vi "Aeroflex ATT Initialize.vi"(8 "error in (no error)":errorcluster, 11 "Configuration":T2={"BusType"=enum."USB", "Card"=0, "USB"="", "IP"=0, "COM"=1, "Baud Rate"=enum."9600"}) -> (0 "error out":errorcluster {"code" format="%.0x"}, 3 "DAQmx Dev Name (PAModule)":string, 5 "Aeroflex ATT":T1)   [LabVIEW 2011]
uses:
  TypeDefs/Aeroflex ATT Configuration.ctl
  TypeDefs/Aeroflex ATT Instrument Info.ctl
  BPIMCore EXT/WebEngine/LIB/MODULES/PA Module/PA Module Tasks.ctl
  <vilib>/DAQmx/create/channels.llb/DAQmx Create Channel (DO-Digital Output).vi
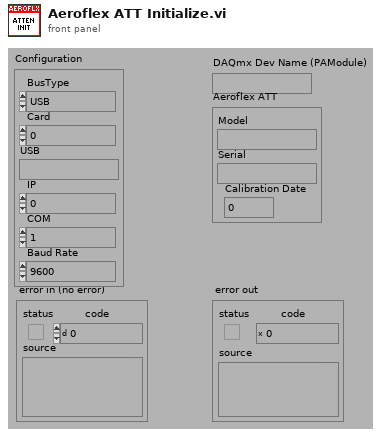
[diagram p1: front panel]
types:
  T1 = typedef "Aeroflex ATT Instrument Info.ctl" = cluster{"Model":string, "Serial":string, "Calibration Date":dbl}
  T2 = typedef "Aeroflex ATT Configuration.ctl" = cluster{"BusType":enum32{"PCI/ISA/PCMCIA", "USB", "Ethernet", "Serial"}, "Card":i32, "USB":string, "IP":u32, "COM":i32, "Baud Rate":enum16{"300", "600", "1200", "2400", "4800", "9600"}}
  T3 = typedef "PA Module Tasks.ctl" = enum16{"PAModule_ID", "PAModule_Alarm", "PAModule_VA1", "PAModule_VA2", "PAModule_SW"}
  T4 = enum32{"PCI/ISA/PCMCIA", "USB", "Ethernet", "Serial"}
  T5 = enum16{"300", "600", "1200", "2400", "4800", "9600"}
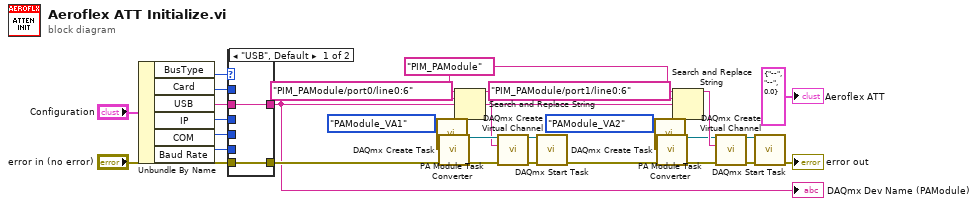
[diagram p0: block diagram]
diagram:
  w1 = "PIM_PAModule" ("DAQmx Dev Name (PIM_PAModule)")
  n1 = Unbundle By Name("Configuration") -> ("BusType"=w29:T4, "Card"=w28:i32, "USB"=w27:string, "IP"=w26:u32, "COM"=w25:i32, "Baud Rate"=w23:T5)
  n2 = case shown="\"USB\", Default" w29 {
    tunnel: "error in (no error)" -> [w32 w33]
    tunnel: w28 -> [_ _]
    tunnel: w27 -> [w31 _]
    tunnel: w26 -> [_ _]
    tunnel: w25 -> [_ _]
    tunnel: [w32 w33] -> w14
    tunnel: [w31 _] -> w4
    tunnel: w23 -> [_ _]
    frame "USB", Default {
    }
    frame "PCI/ISA/PCMCIA", "Ethernet", "Serial" {
    }
  }
  "DAQmx Dev Name (PAModule)" <- w4
  n3 = call "PA Module Task Converter.vi"("PA Module Task"=PA_Module_Tasks."PAModule_VA1" ("RFModule Tasks and Channels")) -> ("Task/Channel Name"=w17:refnum<k21>)  [unwired: 7 out]
  n4 = call <vilib>:"DAQmx Create Task.vi"("new task name"=w17, "error in"=w14) -> ("task out"=w21:refnum<k21>, "error out"=w22:errorcluster)  [unwired: 3 in, 9 out]
  n5 = Search and Replace String(input string=tag "PIM_PAModule/port0/line0:6" ("lines"), search string=w1, replace string=w4) -> (result string=w16:string)  [unwired: 2 in, 6 out]
  n6 = call-poly <vilib>:"DAQmx Create Virtual Channel.vi"("task in"=w21, "lines"=w16, "error in"=w22) -> ("task out"=w19:refnum<k21>, "error out"=w20:errorcluster)  [unwired: 2 in, 9 out]
  n7 = call <vilib>:"DAQmx Start Task.vi"("task/channels in"=w19, "error in"=w20) -> ("error out"=w3:errorcluster)  [unwired: 13 out]
  n8 = call "PA Module Task Converter.vi"("PA Module Task"=PA_Module_Tasks."PAModule_VA2" ("RFModule Tasks and Channels")) -> ("Task/Channel Name"=w10:refnum<k21>)  [unwired: 7 out]
  n9 = call <vilib>:"DAQmx Create Task.vi"("new task name"=w10, "error in"=w3) -> ("task out"=w6:refnum<k21>, "error out"=w5:errorcluster)  [unwired: 3 in, 9 out]
  n10 = Search and Replace String(input string=tag "PIM_PAModule/port1/line0:6" ("lines"), search string=w1, replace string=w4) -> (result string=w11:string)  [unwired: 2 in, 6 out]
  n11 = call-poly <vilib>:"DAQmx Create Virtual Channel.vi"("task in"=w6, "lines"=w11, "error in"=w5) -> ("task out"=w8:refnum<k21>, "error out"=w7:errorcluster)  [unwired: 2 in, 9 out]
  n12 = call <vilib>:"DAQmx Start Task.vi"("task/channels in"=w8, "error in"=w7) -> ("error out"=→"error out":errorcluster)  [unwired: 13 out]
  "Aeroflex ATT" <- T1 {"Model"="--", "Serial"="--", "Calibration Date"=0.0} ("Aeroflex ATT")
